vi "Configure Pulse.vi"(0 "VISA resource name":refnum<visa-resource-name>, 1 "Duty (20%)":dbl=20.0 min=0.0001 max=100.0 format="%.4g", 5 "Channel (1:Channel 1)":i32(ring)=1 items=["Channel 1"=1, "Channel 2"=2], 7 "Delay (0.00 s)":dbl min=-1000000.0 max=1000000.0, 9 "Rise (20 ns)":dbl=2e-08 format="%#.3g", 11 "error in (no error)":errorcluster, 12 "Fall (20 ns)":dbl=2e-08 format="%#.3g") -> (4 "VISA resource name out":refnum<visa-resource-name>, 15 "error out":errorcluster)   [LabVIEW 2023, in "Siglent SDG X Series.lvlib"]
doc: "Configures the pulse waveform and parameters."
uses:
  Siglent SDG X Series.lvlib
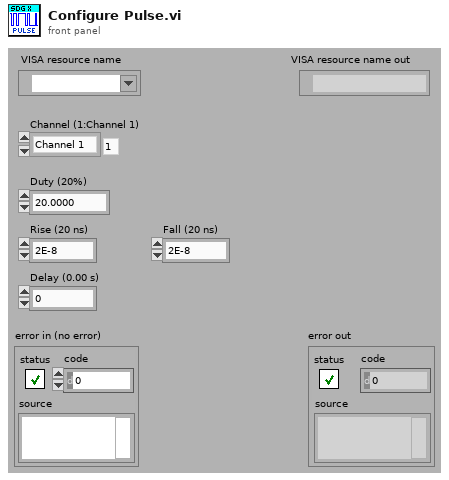
[diagram p1: front panel]
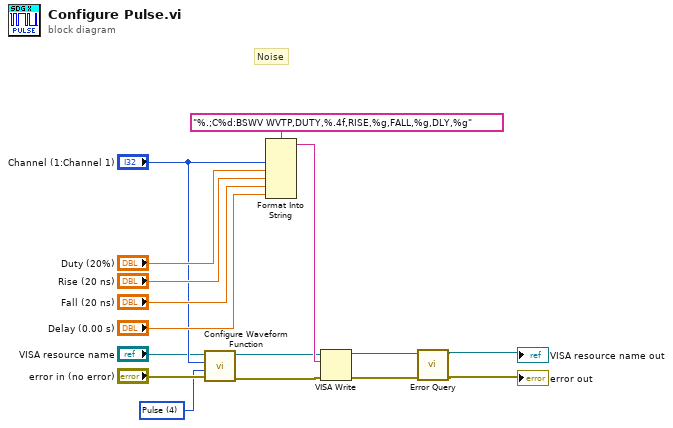
[diagram p0: block diagram]
diagram:
  w1 = u16 4 items=["Sine", "Square", "Ramp", "DC", "Pulse", "Arb", "Noise", "PRBS", "IQ"] ("Waveform Function (0: Sine)")
  # "Noise"
  n1 = call "Configure Waveform Function.vi"("error in (no error)"="error in (no error)", "Waveform Function (0: Sine)"=w1, "Channel (1:Channel 1)"="Channel (1:Channel 1)", "VISA resource name"="VISA resource name") -> ("error out"=w3:errorcluster, "VISA resource name out"=w2:refnum<visa-resource-name>)  [unwired: 6 in]
  n2 = Format Into String(format string="%.;C%d:BSWV WVTP,DUTY,%.4f,RISE,%g,FALL,%g,DLY,%g", "Channel (1:Channel 1)", "Duty (20%)", "Rise (20 ns)", "Fall (20 ns)", "Delay (0.00 s)") -> (resulting string=w15:string)  [unwired: 2 in, 1 out]
  n3 = VISA Write(VISA resource name=w2, write buffer=w15, error in (no error)=w3) -> (VISA resource name out=w10:refnum<visa-resource-name>, error out=w9:errorcluster)  [unwired: 1 out]
  n4 = call "Error Query.vi"("error in (no error)"=w9, "VISA resource name"=w10) -> ("error out"=→"error out":errorcluster, "VISA resource name out"=→"VISA resource name out":refnum<visa-resource-name>)  [unwired: 6 in, 2 out]
